vi "Read PV URL.vi"(8 "error in (no error)":errorcluster, 11 "PVConnection in":refnum<class "PVConnection.lvclass">) -> (0 "error out":errorcluster, 2 "PV URL":string, 3 "PVConnection out":refnum<class "PVConnection.lvclass">)   [LabVIEW 2013, in "CS++ProcessVariables.lvlib" / "PVConnection.lvclass"]
uses:
  PVConnection.lvclass
  PVConnection.lvclass/PVConnection.ctl
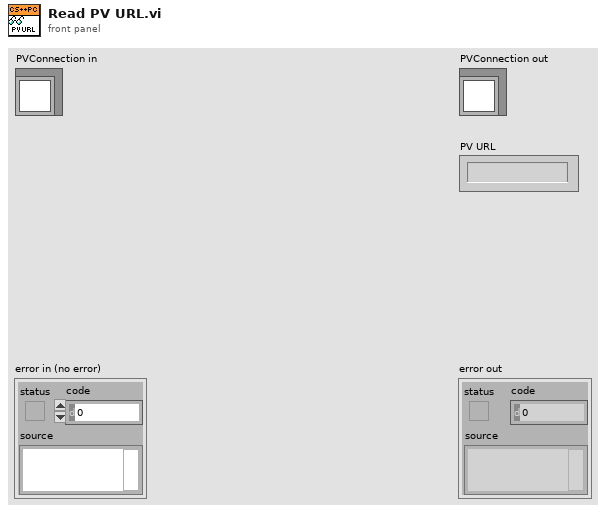
[diagram p1: front panel]
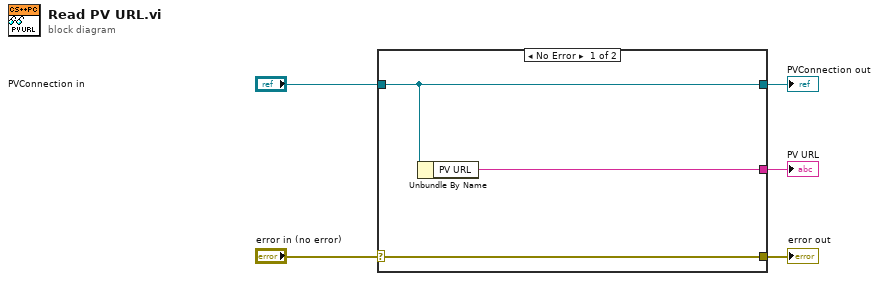
[diagram p0: block diagram]
diagram:
  n1 = case shown="No Error" "error in (no error)" {
    selector: "error in (no error)" -> [w8 w9]
    tunnel: [w8 w9] -> w4
    tunnel: [w7 w10] -> w2
    tunnel: "PVConnection in" -> [w7 w10]
    tunnel: [w6 _] -> w1
    frame No Error {
      n2 = Unbundle By Name(w7) -> ("PV URL"=w6:string)
    }
    frame Error {
    }
  }
  "error out" <- w4
  "PVConnection out" <- w2
  "PV URL" <- w1
